vi "Sub_resample.vi"(11 "Experiment in":T1) -> (3 "Experiment":T1)   [LabVIEW 2021]
panel:
  out "old signal length":i32
  out "new signal length":i32
  out "Resampled Signal":dbl[](graph)
  out "Original signal":dbl[](graph)
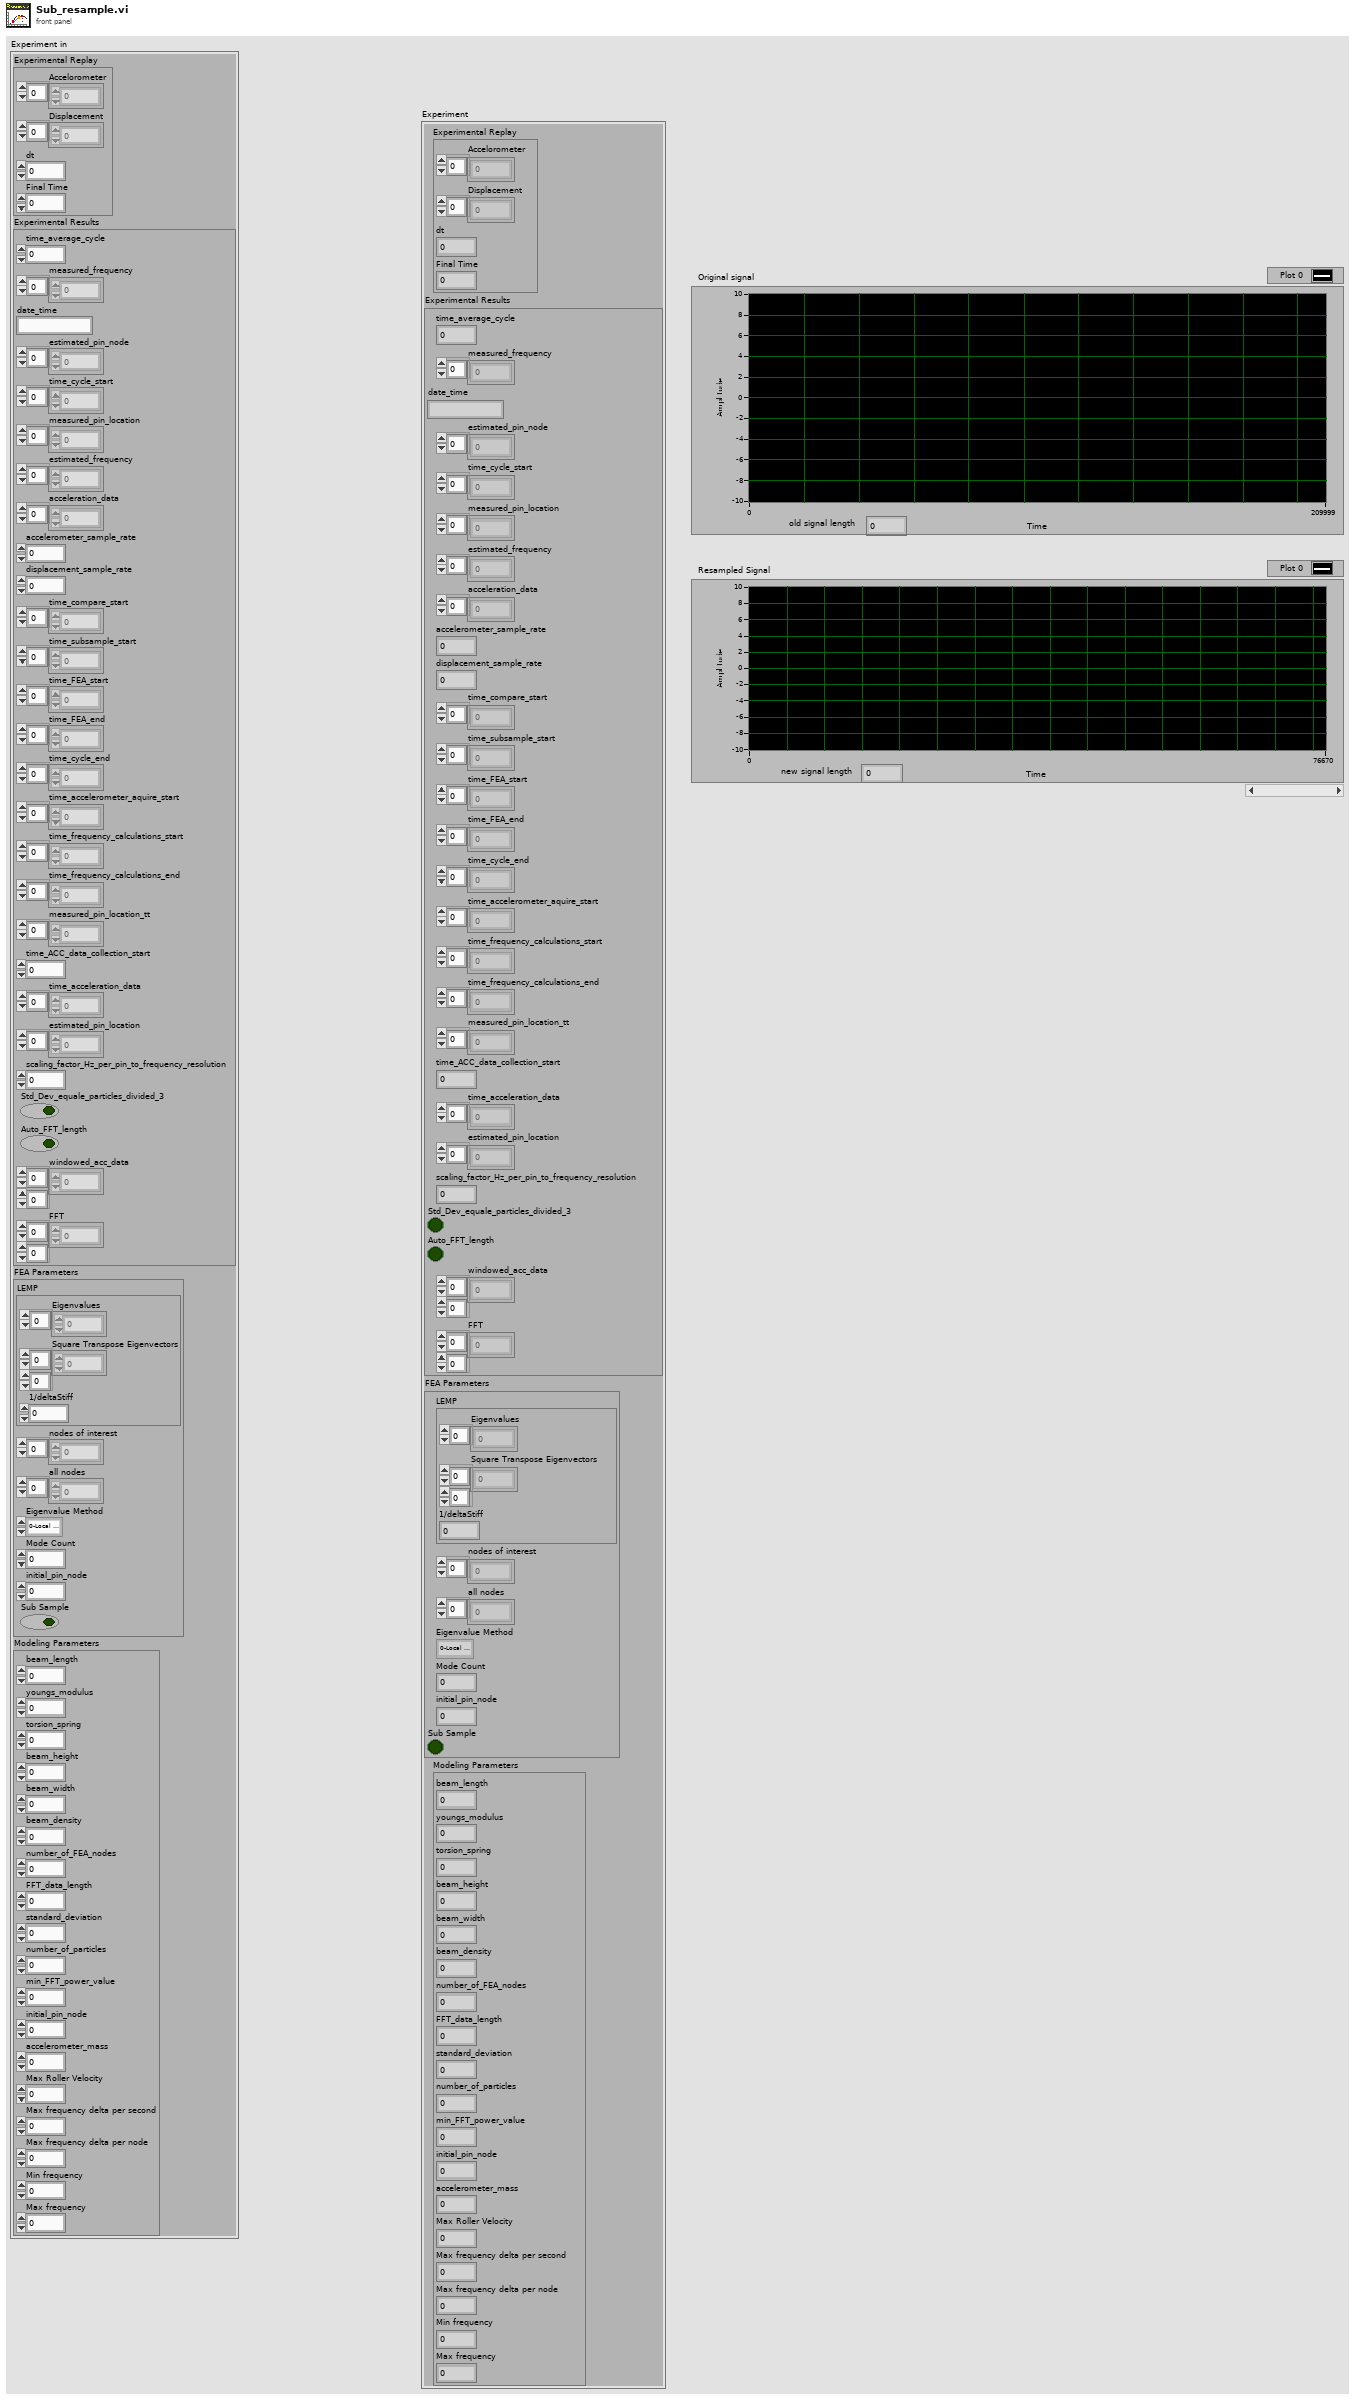
[diagram p1: front panel]
types:
  T1 = cluster{"Experimental Replay":cluster{"Accelorometer":dbl[], "Displacement":dbl[], "dt":dbl, "Final Time":dbl}, "Experimental Results":cluster{"time_average_cycle":dbl, "measured_frequency":dbl[], "date_time":string, "estimated_pin_node":i32[], "time_cycle_start":dbl[], "measured_pin_location":dbl[], "estimated_frequency":dbl[], "acceleration_data":dbl[], "accelerometer_sample_rate":dbl, "displacement_sample_rate":dbl, "time_compare_start":dbl[], "time_subsample_start":dbl[], "time_FEA_start":dbl[], "time_FEA_end":dbl[], "time_cycle_end":dbl[], "time_accelerometer_aquire_start":dbl[], "time_frequency_calculations_start":dbl[], "time_frequency_calculations_end":dbl[], "measured_pin_location_tt":dbl[], "time_ACC_data_collection_start":dbl, "time_acceleration_data":dbl[], "estimated_pin_location":dbl[], "scaling_factor_Hz_per_pin_to_frequency_resolution":dbl, "Std_Dev_equale_particles_divided_3":bool, "Auto_FFT_length":bool, "windowed_acc_data":dbl[][], "FFT":dbl[][]}, "FEA Parameters":cluster{"LEMP":cluster{"Eigenvalues":dbl[], "Square Transpose Eigenvectors":dbl[][], "1/deltaStiff":dbl}, "nodes of interest":i32[], "all nodes":i32[], "Eigenvalue Method":enum16{"0-Local Eigen Modification Procedure", "1-LabVIEW generalized eigenvalues", "2-LabVIEW M^-1K eigenvalues", "3-LabVIEW Cholesky Factorization", "4-Cholesky Factorization CPU SGL", "5-Cholesky Factorization CPU FXP", "6-Cholesky Factorization FPGA SGL", "7-Cholesky Factorization FPGA SGL SCL"}, "Mode Count":i32, "initial_pin_node":i32, "Sub Sample":bool}, "Modeling Parameters":cluster{"beam_length":dbl, "youngs_modulus":dbl, "torsion_spring":dbl, "beam_height":dbl, "beam_width":dbl, "beam_density":dbl, "number_of_FEA_nodes":i32, "FFT_data_length":i32, "standard_deviation":dbl, "number_of_particles":i32, "min_FFT_power_value":dbl, "initial_pin_node":i32, "accelerometer_mass":dbl, "Max Roller Velocity":dbl, "Max frequency delta per second":dbl, "Max frequency delta per node":dbl, "Min frequency":dbl, "Max frequency":dbl}}
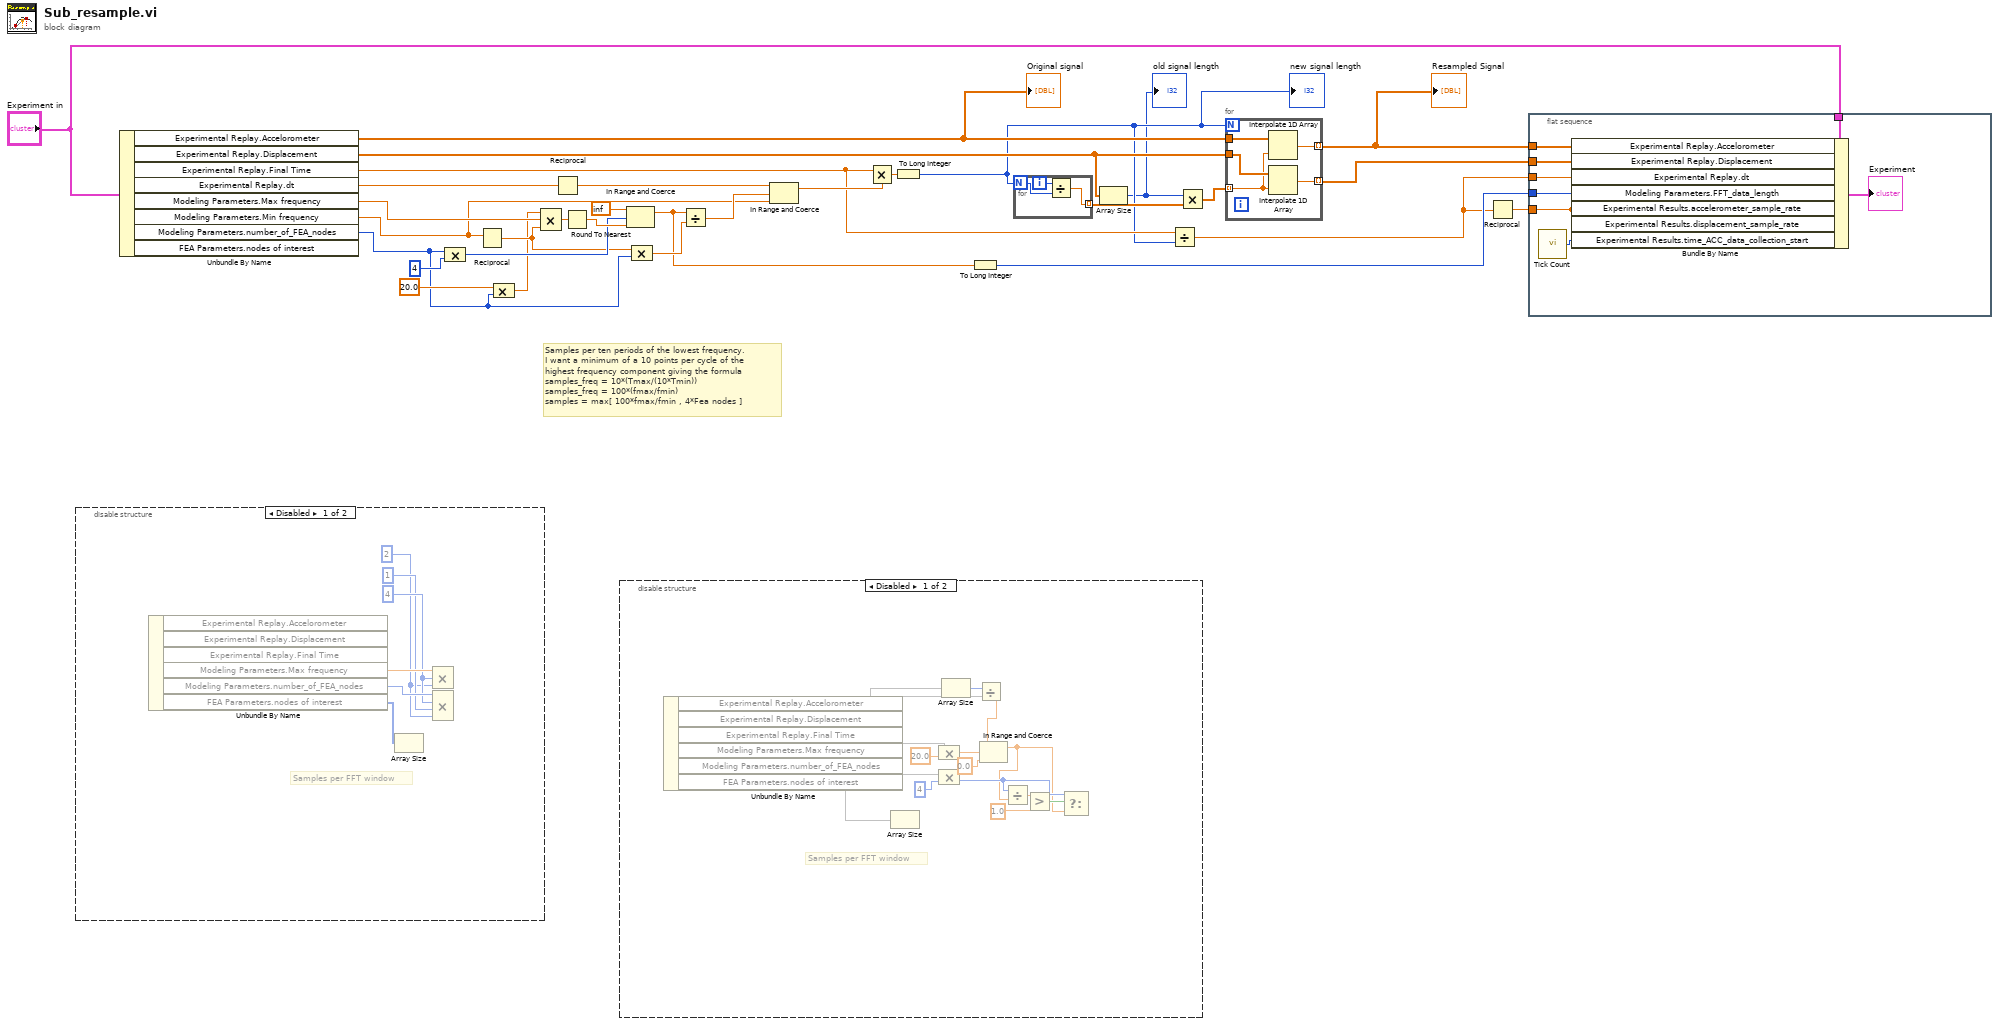
[diagram p0: block diagram]
diagram:
  # "Samples per ten periods of the lowest frequency. \nI want a minimum of a 10 points per cycle of the \nhighest frequency component giving the formula\nsamples_freq = 10*(Tmax/(10*Tmin)) \nsamples_freq = 100*(fmax/fmin)\nsamples = max[ 100*fmax/fmin , 4*Fea nodes ]"
  n1 = disable-structure shown="Disabled" {
    frame Disabled {
      w32 = 2
      w34 = 4 ("y")
      # "Samples per FFT window"
      n2 = Unbundle By Name() -> ("Experimental Replay.Final Time"=w39:dbl, "Modeling Parameters.Max frequency"=w35:dbl, "Modeling Parameters.number_of_FEA_nodes"=w36:i32, "FEA Parameters.nodes of interest"=w38:i32[])  [unwired: 1 in, 2 out]
      n3 = Array Size(array=w38) -> (size(s)=w37:i32)
      n4 = Compound Arithmetic op=MULTIPLY(w35, w34, w32) -> ()  [unwired: 1 out]
      n5 = Compound Arithmetic op=MULTIPLY(w36, w34, 1 ("y"), w32) -> ()  [unwired: 1 out]
    }
    frame Enabled {
    }
  }
  n6 = Unbundle By Name("Experiment in") -> ("Experimental Replay.Accelorometer"=w13:dbl[], "Experimental Replay.Displacement"=w12:dbl[], "Experimental Replay.Final Time"=w8:dbl, "Experimental Replay.dt"=w11:dbl, "Modeling Parameters.Max frequency"=w22:dbl, "Modeling Parameters.Min frequency"=w15:dbl, "Modeling Parameters.number_of_FEA_nodes"=w3:i32)  [unwired: 1 out]
  "Original signal" <- w13
  n7 = Compound Arithmetic op=MULTIPLY(w3, 4 ("Modeling Parameters.number_of_FEA_nodes")) -> (w19:i32)
  n8 = Reciprocal(x=w15) -> (1/x=w18:dbl)
  n9 = Compound Arithmetic op=MULTIPLY(20.0 ("value"), w3) -> (w4:dbl)
  n10 = Compound Arithmetic op=MULTIPLY(w4, w22, w18) -> (w21:dbl)
  n11 = Reciprocal(x=w11) -> (1/x=w10:dbl)
  n12 = Round To Nearest(number=w21) -> (nearest integer value=w20:dbl)
  n13 = disable-structure shown="Disabled" {
    frame Disabled {
      # "Samples per FFT window"
      n14 = Unbundle By Name() -> (w56:T1, "Experimental Replay.Accelorometer"=w48, "Experimental Replay.Final Time"=w46, "Modeling Parameters.Max frequency"=w54, "Modeling Parameters.number_of_FEA_nodes"=w53, "FEA Parameters.nodes of interest"=w55)  [unwired: 1 out]
      n15 = Array Size(array=w55) -> ()  [unwired: 1 out]
      n16 = Compound Arithmetic op=MULTIPLY(w54, 20.0 ("value")) -> (w49:dbl)
      n17 = Compound Arithmetic op=MULTIPLY(w53, 4 ("y")) -> (w43:i32)
      n18 = Array Size(array=w48) -> (size(s)=w47:i32)
      n19 = Divide(x=w47, y=w46) -> (x/y=w45:dbl)
      n20 = In Range and Coerce(upper limit=w45, x=w49, lower limit=0.0 ("result")) -> (coerced(x)=w42:dbl)  [unwired: 1 out]
      n21 = Divide(x=w43, y=w42) -> (x/y=w51:dbl)
      n22 = Greater?(x=w51, y=1.0) -> (0:w52:bool)
      n23 = Select(t=w43, s=w52, f=w42) -> ()  [unwired: 1 out]
    }
    frame Enabled {
    }
  }
  n24 = In Range and Coerce(upper limit=inf, x=w19, lower limit=w20) -> (coerced(x)=w14:dbl)  [unwired: 1 out]
  n25 = Compound Arithmetic op=MULTIPLY(w18, w3) -> (w17:dbl)
  n26 = Divide(x=w14, y=w17) -> (x/y=w16:dbl)
  n27 = In Range and Coerce(upper limit=w10, x=w16, lower limit=w15) -> (coerced(x)=w9:dbl)  [unwired: 1 out]
  n28 = Multiply(x=w8, y=w9) -> (x*y=w29:dbl)
  n29 = To Long Integer(number=w29) -> (32bit integer=w2:i32)
  "new signal length" <- w2
  n30 = To Long Integer(number=w14) -> (32bit integer=w27:i32)
  n31 = for {
    N: w2 -> [w58]
    tunnel: [w57] -> w31 mode=indexing
    i -> [w59]
    n32 = Divide(x=w59, y=w58) -> (x/y=w57:dbl)
  }
  n33 = Array Size(array=w12) -> (size(s)=w1:i32)
  "old signal length" <- w1
  n34 = Divide(x=w8, y=w2) -> (x/y=w26:dbl)
  n35 = Multiply(x=w1, y=w31) -> (x*y=w30:dbl[])
  n36 = for {
    N: w2 -> [_]
    tunnel: w13 -> [w64]
    tunnel: w12 -> [w63]
    tunnel: w30 -> [w62] mode=indexing
    tunnel: [w61] -> w23 mode=indexing
    tunnel: [w60] -> w24 mode=indexing
    n37 = Interpolate 1D Array(1:w62, 2:w64) -> (0:w61:dbl)
    n38 = Interpolate 1D Array(1:w62, 2:w63) -> (0:w60:dbl)
  }
  "Resampled Signal" <- w23
  n39 = Reciprocal(x=w26) -> (1/x=w25:dbl)
  n40 = flat-sequence {
    tunnel: "Experiment in" -> [w72]
    tunnel: w27 -> [w71]
    tunnel: w24 -> [w70]
    tunnel: w23 -> [w69]
    tunnel: w26 -> [w67]
    tunnel: w25 -> [w66]
    frame #0 {
      n41 = call "Tick Count"() -> ("Tick Count(uSec)"=w65:u32)
      n42 = Bundle By Name(cluster=w72, "Experimental Replay.Accelorometer"=w69, "Experimental Replay.Displacement"=w70, "Experimental Replay.dt"=w67, "Modeling Parameters.FFT_data_length"=w71, "Experimental Results.accelerometer_sample_rate"=w66, "Experimental Results.displacement_sample_rate"=w66, "Experimental Results.time_ACC_data_collection_start"=w65) -> (→"Experiment":T1)
    }
  }
